vi "subtract.vi"(10 "Numeric 4":dbl, 11 "Numeric 3":dbl) -> (1 "A+B 3":bool[][](array[boolean]), 2 "negative":bool, 3 "A 2":bool[](array[boolean]), 4 "B 2":bool[](array[boolean]), 5 "A+B 2":dbl)   [LabVIEW 2020]
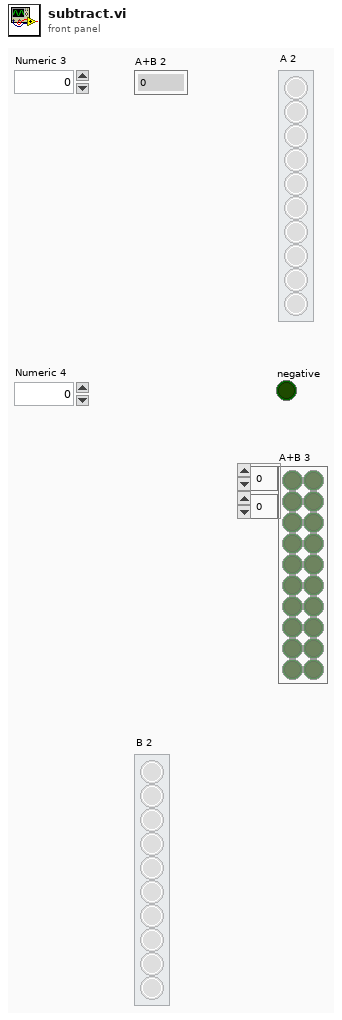
[diagram p1: front panel]
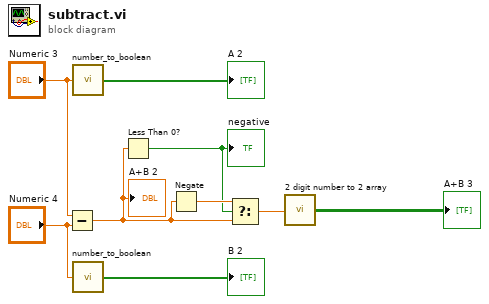
[diagram p0: block diagram]
diagram:
  n1 = Subtract(x="Numeric 3", y="Numeric 4") -> (x-y=w9:dbl)
  "A+B 2" <- w9
  n2 = call "number_to_boolean.vi"("A in"="Numeric 3") -> ("A out"=→"A 2":bool[])
  n3 = call "number_to_boolean.vi"("A in"="Numeric 4") -> ("A out"=→"B 2":bool[])
  n4 = Less Than 0?(x=w9) -> (x < 0?=w5:bool)
  "negative" <- w5
  n5 = Negate(x=w9) -> (-x=w8:dbl)
  n6 = Select(t=w8, s=w5, f=w9) -> (s? t:f=w7:dbl)
  n7 = call "2 digit number to 2 array.vi"("Numeric"=w7) -> ("transposed array"=→"A+B 3":bool[][])
